vi "Find VI on Disk.vi"(10 "pattern":string, 11 "Directory to search":path) -> (3 "Found":string[](array[string]))   [LabVIEW 2020]
panel:
  in  "Tab Control":enum32{"Page 1", "Page 2"}(tab)
  in  "Search":bool
  out "Current directory/llb":path
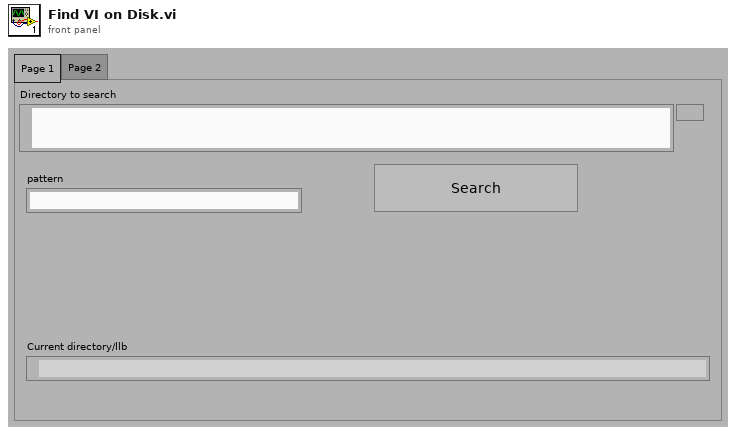
[diagram p1: front panel]
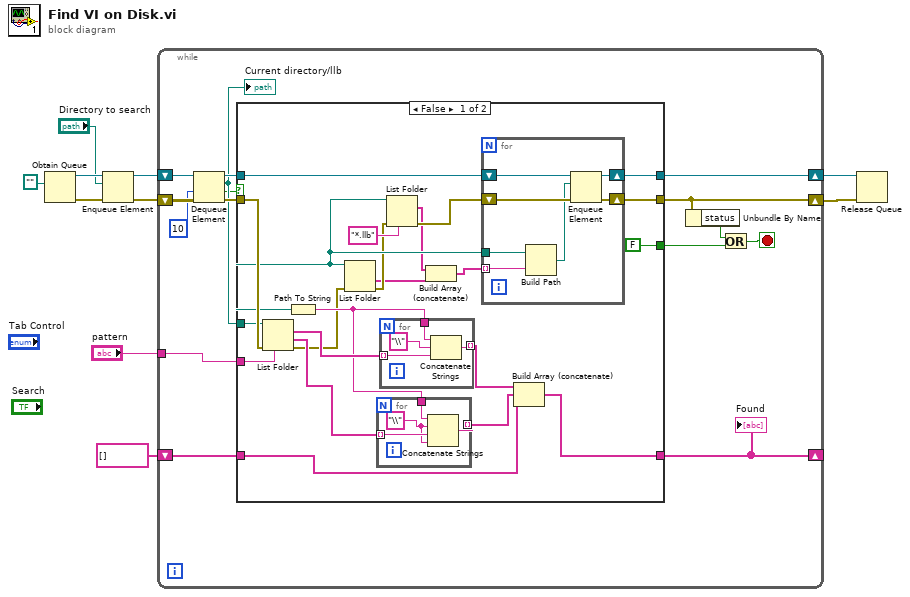
[diagram p0: block diagram]
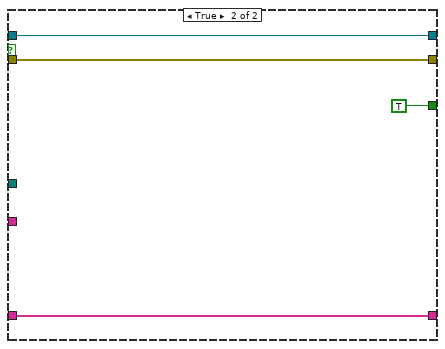
[diagram p2: hidden frame]
diagram:
  n1 = Obtain Queue(element data type=path "") -> (queue out=w9:refnum<queue>, error out=w8:errorcluster)  [unwired: 4 in, 1 out]
  n2 = Enqueue Element(queue=w9, element="Directory to search", error in (no error)=w8) -> (queue out=w6:refnum<queue>, error out=w5:errorcluster)  [unwired: 1 in, 1 out]
  n3 = while {
    shift-right: [w22] -> _
    shift-left: string[] [] ("folder names") -> [w21]
    shift-right: [w19] -> w3
    shift-left: w6 -> [w24]
    shift-right: [w14] -> w2
    shift-left: w5 -> [w25]
    tunnel: "pattern" -> [w16]
    stop <- w12 stop-if-true
    n4 = Dequeue Element(queue=w24, timeout in ms (-1)=10, error in (no error)=w25) -> (queue out=w20:refnum<queue>, element=w17:path, timed out?=w15:bool, error out=w18:errorcluster)
    "Current directory/llb" <- w17
    n5 = case shown="False" w15 {
      tunnel: [w45 w63] -> w22
      tunnel: w21 -> [w40 w63]
      tunnel: w20 -> [w38 w65]
      tunnel: [w37 w65] -> w19
      tunnel: w18 -> [w36 w64]
      tunnel: [w35 w64] -> w14
      tunnel: w17 -> [w34 _]
      tunnel: w16 -> [w27 _]
      tunnel: [FALSE TRUE] -> w11
      frame False {
        n6 = List Folder(path=w34, pattern=w27, error in=w36) -> (filenames=w44:string[], folder names=w42:string[], error out=w39:errorcluster)  [unwired: 1 in, 1 out]
        n7 = Path To String(path=w34) -> (string=w43:string)
        n8 = List Folder(path=w34, error in=w39) -> (folder names=w30:string[], error out=w31:errorcluster)  [unwired: 2 in, 2 out]
        n9 = for {
          tunnel: w43 -> [w57]
          tunnel: w42 -> [w56] mode=indexing
          tunnel: [w55] -> w41 mode=indexing
          w54 = "\\"
          n10 = Concatenate Strings(w57, w54, w56, w54) -> (w55:string)
        }
        n11 = for {
          tunnel: w43 -> [w61]
          tunnel: w44 -> [w60] mode=indexing
          tunnel: [w58] -> w46 mode=indexing
          n12 = Concatenate Strings(w61, "\\", w60) -> (w58:string)
        }
        n13 = List Folder(path=w34, pattern="*.llb", error in=w31) -> (filenames=w29:string[], error out=w32:errorcluster)  [unwired: 1 in, 2 out]
        n14 = Build Array (concatenate)(w29, w30) -> (w28:string[])
        n15 = for {
          tunnel: w28 -> [w53] mode=indexing
          tunnel: w34 -> [w52]
          shift-right: [w48] -> w35
          shift-left: w32 -> [w51]
          shift-right: [w47] -> w37
          shift-left: w38 -> [w50]
          n16 = Build Path(base path=w52, name or relative path=w53) -> (appended path=w49:path)
          n17 = Enqueue Element(queue=w50, element=w49, error in (no error)=w51) -> (queue out=w47:refnum<queue>, error out=w48:errorcluster)  [unwired: 1 in, 1 out]
        }
        n18 = Build Array (concatenate)(w46, w41, w40) -> (w45:string[])
      }
      frame True {
      }
    }
    "Found" <- w22
    n19 = Unbundle By Name(w14) -> ("status"=w13:bool)
    n20 = Or(x=w13, y=w11) -> (x .or. y?=w12:bool)
  }
  n21 = Release Queue(queue=w3, error in (no error)=w2) -> ()  [unwired: 1 in, 3 out]
